vi "Configure Output.vi"(6 "Trigger Source (0: Immediate)":i32(ring) items=["Immediate", "Triggered"], 8 "error in (no error)":errorcluster, 9 "Voltage Level (0.0 V)":dbl min=0.0 max=600.0 format="%.2g", 10 "Enable Output (T: Enable)":bool=TRUE, 11 "VISA resource name":refnum<visa-resource-name>) -> (0 "error out":errorcluster, 3 "VISA resource name out":refnum<visa-resource-name>)   [LabVIEW 2014, in "Agilent N87XX Series.lvlib"]
doc: "Configures output voltage level and enables or disables the output of the power supply. If you set the level for the triggered state, you can send a trigger with the Send Software Trigger VI."
uses:
  Agilent N87XX Series.lvlib
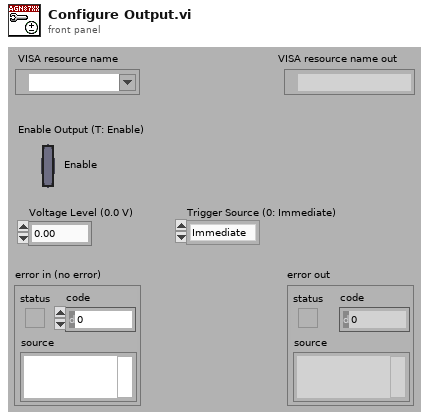
[diagram p1: front panel]
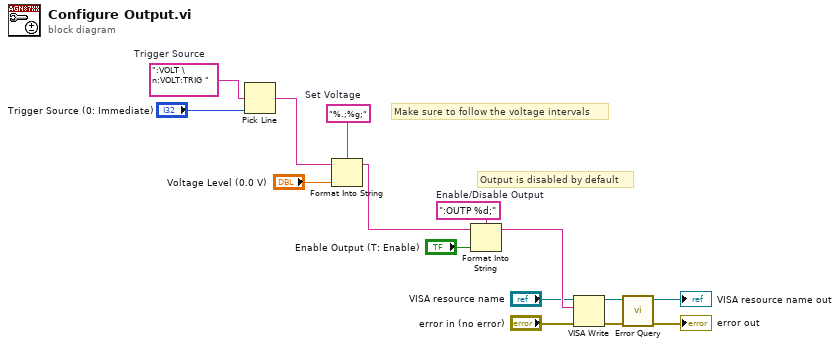
[diagram p0: block diagram]
diagram:
  w4 = ":VOLT \n:VOLT:TRIG "  # Trigger Source
  w12 = ":OUTP %d;"  # Enable/Disable Output
  w1 = "%.;%g;"  # Set Voltage
  # "Make sure to follow the voltage intervals"
  # "Output is disabled by default"
  n1 = Pick Line(multi-line string=w4, line index="Trigger Source (0: Immediate)") -> (output string=w2:string)  [unwired: 1 in]
  n2 = Format Into String(format string=w1, initial string=w2, "Voltage Level (0.0 V)") -> (resulting string=w8:string)  [unwired: 1 in, 1 out]
  n3 = Format Into String(format string=w12, initial string=w8, "Enable Output (T: Enable)") -> (resulting string=w9:string)  [unwired: 1 in, 1 out]
  n4 = VISA Write(VISA resource name="VISA resource name", write buffer=w9, error in (no error)="error in (no error)") -> (VISA resource name out=w11:refnum<visa-resource-name>, error out=w10:errorcluster)  [unwired: 1 out]
  n5 = call "Error Query.vi"("error in (no error)"=w10, "VISA resource name"=w11) -> ("error out"=→"error out":errorcluster, "VISA resource name out"=→"VISA resource name out":refnum<visa-resource-name>)  [unwired: 6 in, 2 out]
